vi "Sum_Saturate_U32.vi"(8 "Sum In":u32, 11 "New Value":u32) -> (0 "Sum Out":u32)   [LabVIEW 2012]
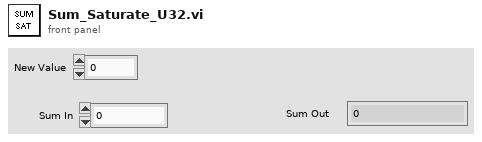
[diagram p1: front panel]
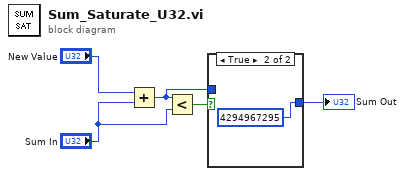
[diagram p0: block diagram]
diagram:
  n1 = Add(x="New Value", y="Sum In") -> (x+y=w2:u32)
  n2 = Less?(x=w2, y="Sum In") -> (x < y?=w4:bool)
  n3 = case shown="True" w4 {
    tunnel: w2 -> [w6 _]
    tunnel: [w6 u32 4294967295] -> w1
    frame False {
    }
    frame True {
    }
  }
  "Sum Out" <- w1
